vi "Example.vi"() -> ()   [LabVIEW 2021]
doc: "Example showing basic usage of the BR_error_handling library. \nTo be able to use this library, it is necessary to initialize error handler first (Init Error Handler.vi), which will search for the XML file in format: '*-errors.txt' with specified custom errors in application directory and its subfolders. \nTo generate custom error, which format is specified in TXT file, use Generate Error.vi and wire required error code to the input with eventual inputs for error description.\nCase structure easily shows multiple use-cases and situations that can occure during using this library."
panel:
  out "Generated Error 1":errorcluster
  out "Generated Error 7":errorcluster
  out "Generated Error 6":errorcluster
  out "Generated Error 5":errorcluster
  out "Generated Error 2":errorcluster
  out "Generated Error 4":errorcluster
  out "Generated Error 3":errorcluster
  # "Overview: Demonstrates how the error_handling library works, and how to wire inputs to Generate Error function. \nInstructions:\n1. Examine the different cases in the block diagram, showing different methods of wiring inputs to error message.\n2. Select the case to be executed from Error format type enum.\n3. Run the VI."
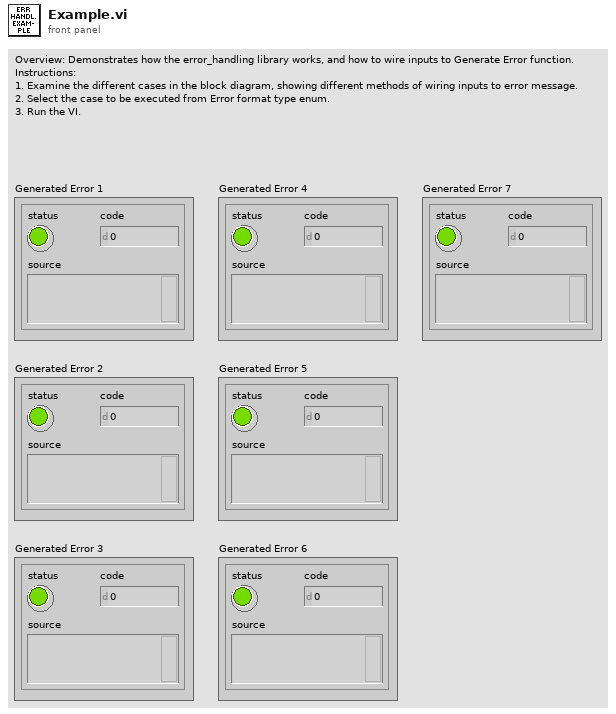
[diagram p1: front panel]
types:
  T1 = cluster{string, i32[], cluster{dbl, bool, i32[]}}
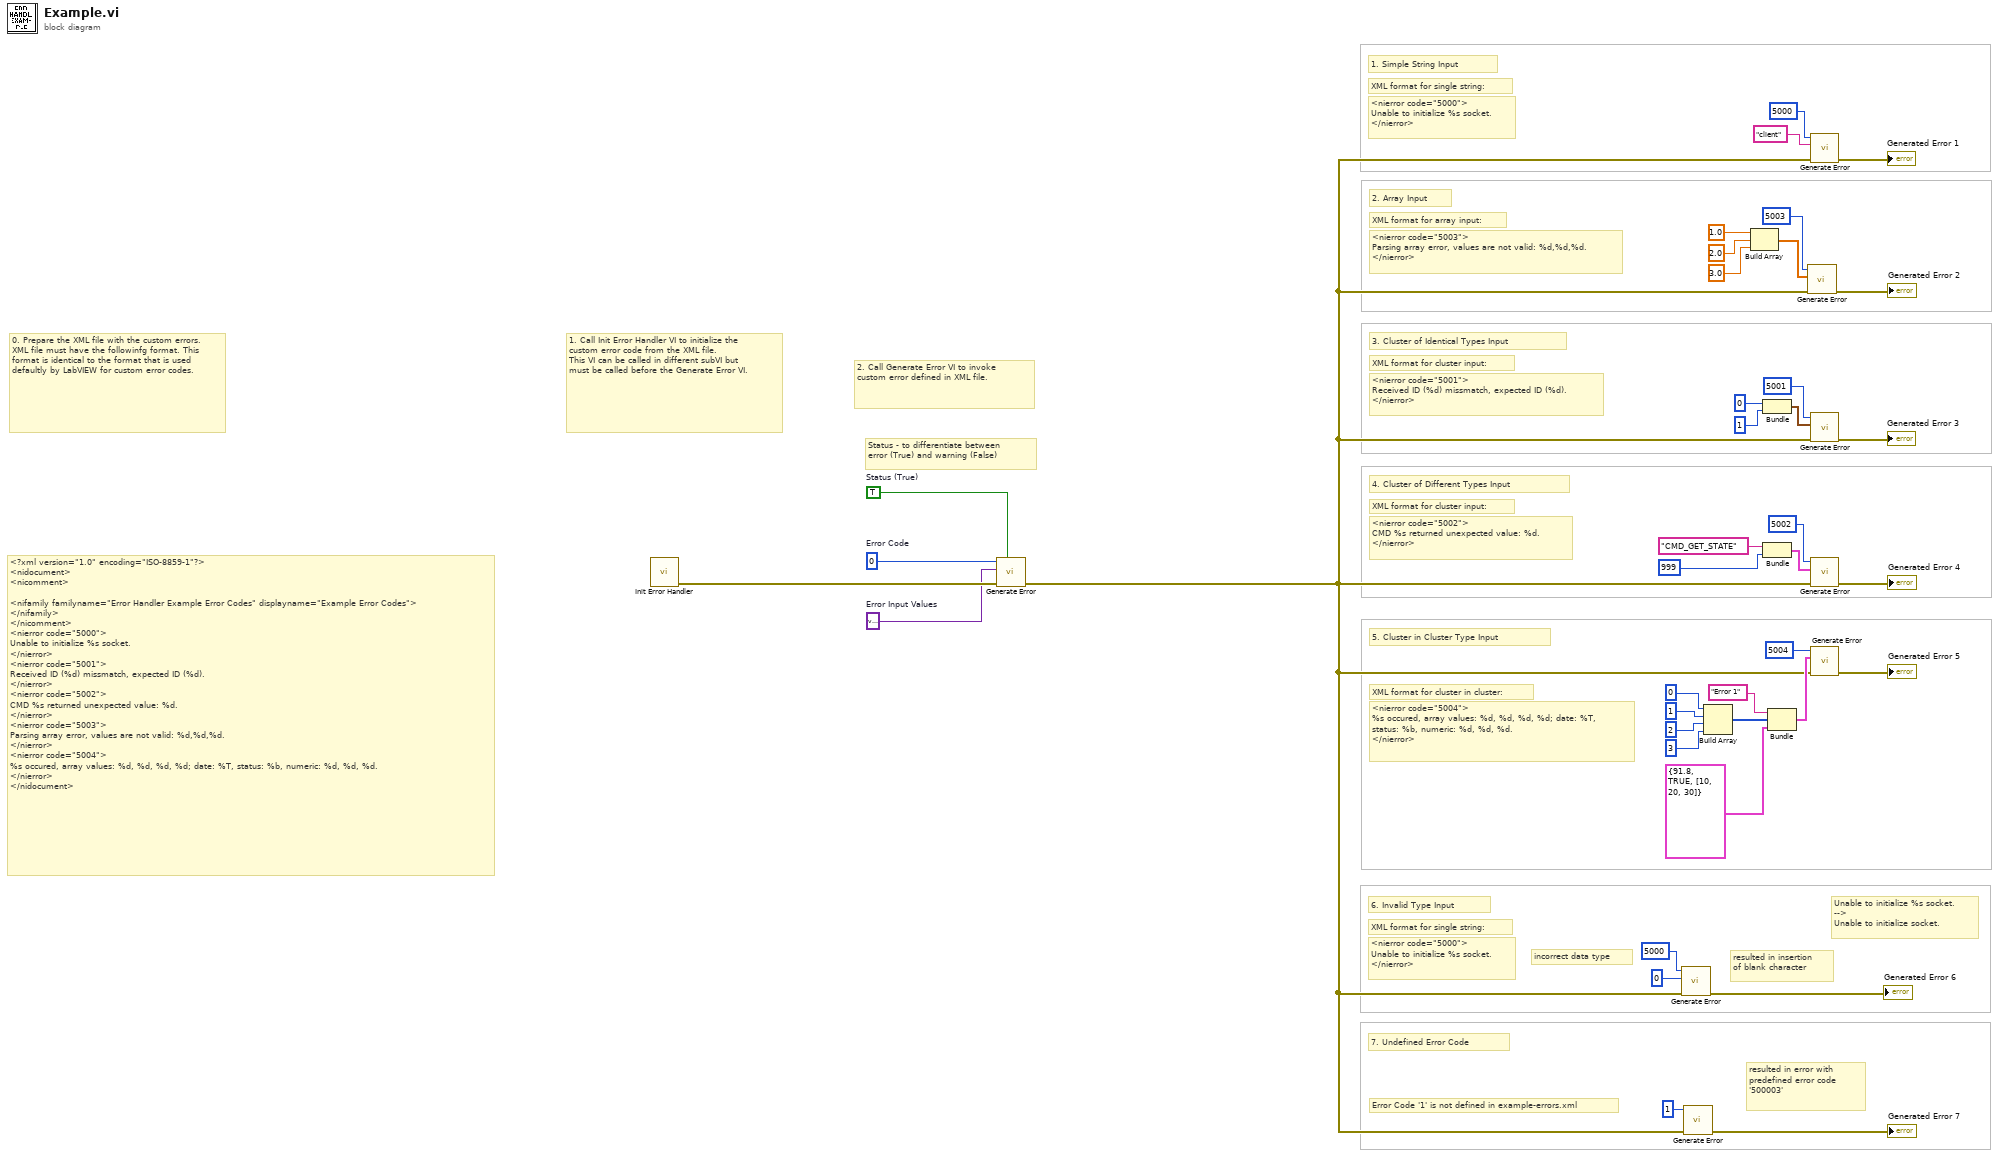
[diagram p0: block diagram]
diagram:
  w1 = variant  # Error Input Values
  w2 = 0  # Error Code
  w3 = TRUE  # Status (True)
  # "Status - to differentiate between error (True) and warning (False)"
  # "<?xml version=\"1.0\" encoding=\"ISO-8859-1\"?>\n<nidocument>\n<nicomment>\n\n<nifamily familyname=\"Error Handler Example Error Codes\" displayname=\"Example Error Codes\">\n</nifamily>\n</nicomment>\n<nierror code=\"5000\">\nUnable to initialize %s socket.\n</nierror>\n<nierror code=\"5001\">\nReceived ID (%d) missmatch, expected ID (%d).\n</nierror>\n<nierror code=\"5002\">\nCMD %s returned unexpected value: %d.\n</nierror>\n<nierror code=\"5003\">\nParsing array error, values are not valid: %d,%d,%d.\n</nierror>\n<nierror code=\"5004\">\n%s occured, array values: %d, %d, %d, %d; date: %T, status: %b, numeric: %d, %d, %d.\n</nierror>\n</nidocument>"
  # "0. Prepare the XML file with the custom errors. XML file must have the followinfg format. This format is identical to the format that is used defaultly by LabVIEW for custom error codes."
  # "2. Call Generate Error VI to invoke custom error defined in XML file."
  # "1. Call Init Error Handler VI to initialize the custom error code from the XML file. \nThis VI can be called in different subVI but must be called before the Generate Error VI."
  # "resulted in error with predefined error code '500003'"
  # "Error Code '1' is not defined in example-errors.xml"
  # "7. Undefined Error Code"
  # "Unable to initialize %s socket.\n-->\nUnable to initialize socket."
  # "resulted in insertion of blank character"
  # "incorrect data type"
  # "XML format for single string:"
  # "<nierror code=\"5000\">\nUnable to initialize %s socket.\n</nierror>"
  # "6. Invalid Type Input"
  # "XML format for cluster in cluster:"
  # "<nierror code=\"5004\">\n%s occured, array values: %d, %d, %d, %d; date: %T, status: %b, numeric: %d, %d, %d.\n</nierror>"
  # "5. Cluster in Cluster Type Input"
  # "XML format for array input:"
  # "<nierror code=\"5003\">\nParsing array error, values are not valid: %d,%d,%d.\n</nierror>"
  # "2. Array Input"
  # "XML format for cluster input:"
  # "<nierror code=\"5002\">\nCMD %s returned unexpected value: %d.\n</nierror>"
  # "4. Cluster of Different Types Input"
  # "XML format for single string:"
  # "<nierror code=\"5000\">\nUnable to initialize %s socket.\n</nierror>"
  # "1. Simple String Input"
  # "XML format for cluster input:"
  # "<nierror code=\"5001\">\nReceived ID (%d) missmatch, expected ID (%d).\n</nierror>"
  # "3. Cluster of Identical Types Input"
  n1 = call "Init Error Handler.vi"() -> ("error out"=w5:errorcluster)  [unwired: 11 in]
  n2 = call "Generate Error.vi"("Status (True)"=w3, "error in"=w5, "Error Input Values"=w1, "Error Code"=w2) -> ("Generated Error"=w4:errorcluster)  [unwired: 7 in]
  n3 = call "Generate Error.vi"("error in"=w4, "Error Input Values"=0, "Error Code"=5000) -> ("Generated Error"=→"Generated Error 6":errorcluster)  [unwired: 8 in]
  n4 = call "Generate Error.vi"("error in"=w4, "Error Code"=1) -> ("Generated Error"=→"Generated Error 7":errorcluster)  [unwired: 9 in]
  n5 = Build Array(0, 1, 2, 3) -> (w24:i32[])
  n6 = Build Array(1.0, 2.0, 3.0) -> (w29:dbl[])
  n7 = Bundle(0, 1) -> (w37:cluster{i32, i32})  [unwired: 1 in]
  n8 = Bundle("CMD_GET_STATE", 999) -> (w33:cluster{string, i32})  [unwired: 1 in]
  n9 = Bundle("Error 1", w24, cluster{dbl, bool, i32[]} {91.8, TRUE, [10, 20, 30]}) -> (w23:T1)  [unwired: 1 in]
  n10 = call "Generate Error.vi"("error in"=w4, "Error Input Values"=w29, "Error Code"=5003) -> ("Generated Error"=→"Generated Error 2":errorcluster)  [unwired: 8 in]
  n11 = call "Generate Error.vi"("error in"=w4, "Error Input Values"="client", "Error Code"=5000) -> ("Generated Error"=→"Generated Error 1":errorcluster)  [unwired: 8 in]
  n12 = call "Generate Error.vi"("error in"=w4, "Error Input Values"=w37, "Error Code"=5001) -> ("Generated Error"=→"Generated Error 3":errorcluster)  [unwired: 8 in]
  n13 = call "Generate Error.vi"("error in"=w4, "Error Input Values"=w33, "Error Code"=5002) -> ("Generated Error"=→"Generated Error 4":errorcluster)  [unwired: 8 in]
  n14 = call "Generate Error.vi"("error in"=w4, "Error Input Values"=w23, "Error Code"=5004) -> ("Generated Error"=→"Generated Error 5":errorcluster)  [unwired: 8 in]
